vi "Motor_Open.vi"() -> ()   [LabVIEW 2016]
uses:
  <vilib>/Rock Robotics/WPI/SafetyOutput/WPI_SafetyOutputConfigMenu.ctl
  <vilib>/Rock Robotics/SystemInterfaces/DIO/FPGA_DIOPWMChannel.ctl
  <vilib>/Rock Robotics/WPI/ThirdParty/CanMotor/TalonSRX/WPI_CANTalonSRX_APIControlMode.ctl
  Drive/RobotDriveOpen6MotorWithTalonSR.vi
  Drive/RobotDriveOpen6MotorWithTalonSRX.vi
  <vilib>/Rock Robotics/WPI/MotorControl/WPI_MotorControlOpen Talon.vi
panel:
  in  "Left Motor 1 Inverted":bool=TRUE
  in  "Left Motor 2 Inverted":bool=TRUE
  in  "Right Motor 1 Inverted":bool=TRUE
  in  "Right Motor 2 Inverted":bool=TRUE
  in  "Competition_Robot?":bool
  in  "Right Motor 3 Inverted":bool=TRUE
  in  "Right Motor 2 Inverted":bool=TRUE
  in  "Right Motor 1 Inverted":bool=TRUE
  in  "Left Motor 3 Inverted":bool=TRUE
  in  "Left Motor 2 Inverted":bool=TRUE
  in  "Left Motor 1 Inverted":bool=TRUE
  # "Can"
  # "PWM"
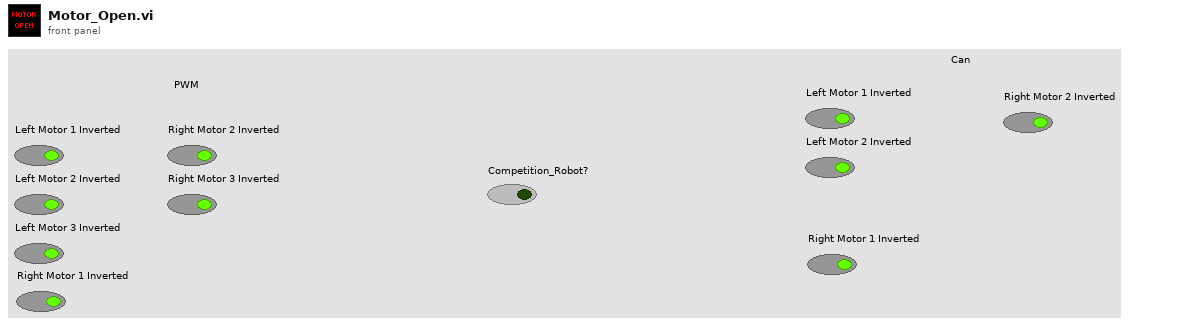
[diagram p1: front panel]
types:
  T1 = typedef "WPI_SafetyOutputConfigMenu.ctl" = enum16{"Enable", "Disable"}
  T2 = typedef "FPGA_DIOPWMChannel.ctl" = enum8{"PWM 0", "PWM 1", "PWM 2", "PWM 3", "PWM 4", "PWM 5", "PWM 6", "PWM 7", "PWM 8", "PWM 9", "PWM MXP 0", "PWM MXP 1", "PWM MXP 2", "PWM MXP 3", "PWM MXP 4", "PWM MXP 5", "PWM MXP 6", "PWM MXP 7", "PWM MXP 8", "PWM MXP 9", "Invalid"}
  T3 = typedef "WPI_CANTalonSRX_APIControlMode.ctl" = enum8{"Percent VBus", "Speed", "Position", "Slave", "Unchanged / Invalid", "Voltage Compensation", "Current", "Motion Profile", "Motion Magic"}
  T4 = typedef "WPI_RobotDriveDevRef.ctl" = cluster{"DevStatus":errorcluster, "Motors[]":T5[], "Square Inputs":bool, "Max Output":dbl}
  T5 = typedef "WPI_MotorControlDeviceRef.ctl" = cluster{"DeviceStatus":errorcluster, "Type":T6, "PWM":cluster{"PWM Channel":T2, "DeadBand":T7}, "CAN":cluster{"Device Number":u8, "SetOutput VI Ref":variant, "GetOutput VI Ref":variant, "Enable VI Ref":variant, "Disable VI Ref":variant, "Data":variant}, "Invert":bool}
  T6 = typedef "WPI_MotorControlType.ctl" = enum16{"PWM", "CAN"}
  T7 = typedef "WPI_PWMDeadband.ctl" = cluster{"Name":string, "maxPositivePwm":i32, "minPositivePwm":i32, "centerPwm":i32, "maxNegativePwm":i32, "minNegativePwm":i32, "angularRange":u16}
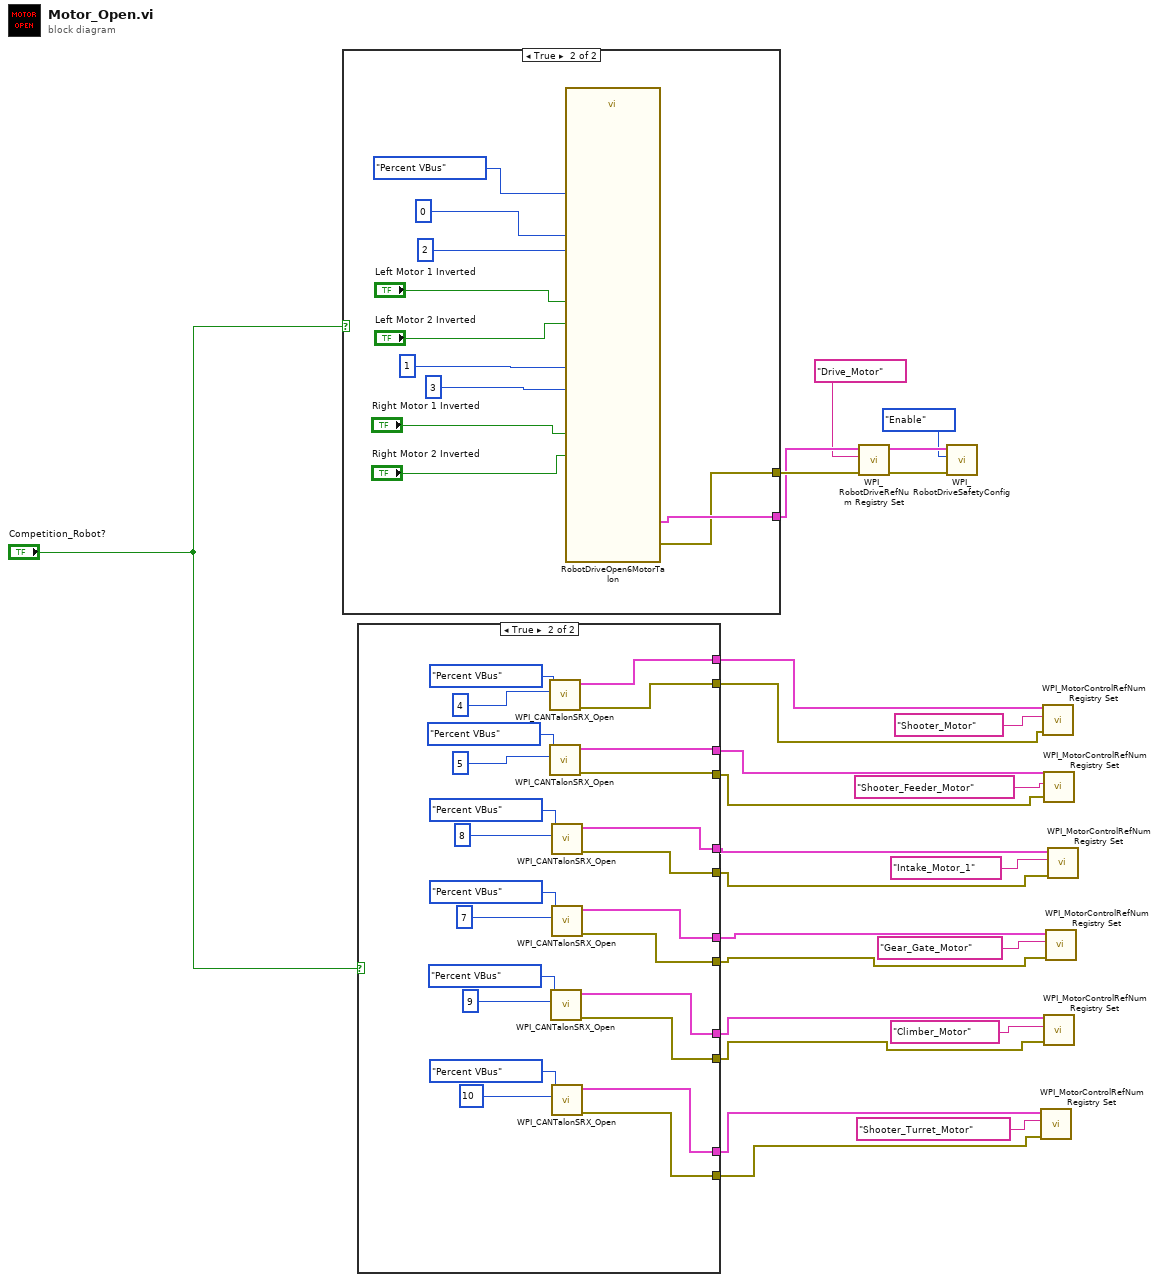
[diagram p0: block diagram]
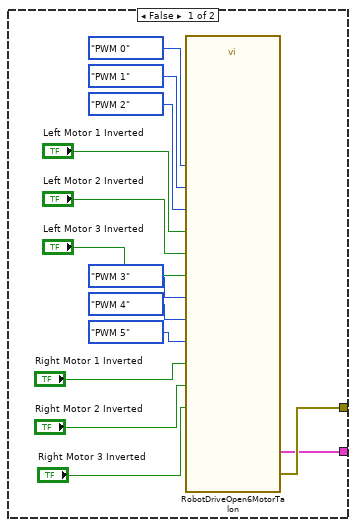
[diagram p2: hidden frame]
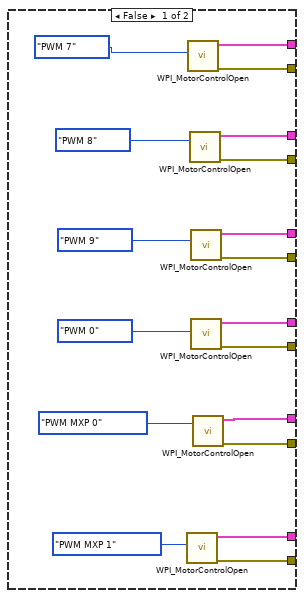
[diagram p3: hidden frame]
diagram:
  n1 = case shown="True" "Competition_Robot?" {
    tunnel: [w33 w45] -> w25
    tunnel: [w32 w46] -> w24
    frame False {
      n2 = call-poly "RobotDriveOpen6MotorTalon.vi"("Left Motor 1"=FPGA_DIOPWMChannel."PWM 0", "Left Motor 2"=FPGA_DIOPWMChannel."PWM 1", "Left Motor 3"=FPGA_DIOPWMChannel."PWM 2", "Right Motor 1"=FPGA_DIOPWMChannel."PWM 3", "Right Motor 2"=FPGA_DIOPWMChannel."PWM 4", "Right Motor 3"=FPGA_DIOPWMChannel."PWM 5", "Left Motor 1 Inverted"="Left Motor 1 Inverted", "Right Motor 1 Inverted"="Right Motor 1 Inverted", "Left Motor 2 Inverted"="Left Motor 2 Inverted", "Right Motor 2 Inverted"="Right Motor 2 Inverted", "Left Motor 3 Inverted"="Left Motor 3 Inverted", "Right Motor 3 Inverted"="Right Motor 3 Inverted") -> ("RobotDriveDevRef"=w32:T4, "error out"=w33:errorcluster)  [unwired: 14 in]
    }
    frame True {
      n3 = call-poly "RobotDriveOpen6MotorTalon.vi"("Left Motor 1"=u8 0, "Left Motor 2"=u8 2, "Right Motor 1"=u8 1, "Right Motor 2"=u8 3, "Left Motor 1 Inverted"="Left Motor 1 Inverted", "Right Motor 1 Inverted"="Right Motor 1 Inverted", "Left Motor 2 Inverted"="Left Motor 2 Inverted", "Right Motor 2 Inverted"="Right Motor 2 Inverted", "Control Mode"=WPI_CANTalonSRX_APIControlMode."Percent VBus") -> ("RobotDriveDevRef"=w46:T4, "error out"=w45:errorcluster)  [unwired: 17 in]
    }
  }
  n4 = case shown="True" "Competition_Robot?" {
    tunnel: [w62 w80] -> w13
    tunnel: [w61 w79] -> w12
    tunnel: [w60 w78] -> w11
    tunnel: [w59 w77] -> w10
    tunnel: [w58 w76] -> w9
    tunnel: [w57 w75] -> w8
    tunnel: [w56 w74] -> w7
    tunnel: [w55 w73] -> w6
    tunnel: [w54 w72] -> w5
    tunnel: [w53 w71] -> w4
    tunnel: [w52 w70] -> w3
    tunnel: [w51 w69] -> w2
    frame False {
      n5 = call-poly <vilib>:"WPI_MotorControlOpen.vi"("PWM Channel"=FPGA_DIOPWMChannel."PWM MXP 1") -> ("error out"=w51:errorcluster, "MotorControlDeviceRef"=w52:T5)  [unwired: 9 in]
      n6 = call-poly <vilib>:"WPI_MotorControlOpen.vi"("PWM Channel"=FPGA_DIOPWMChannel."PWM 7") -> ("error out"=w61:errorcluster, "MotorControlDeviceRef"=w62:T5)  [unwired: 9 in]
      n7 = call-poly <vilib>:"WPI_MotorControlOpen.vi"("PWM Channel"=FPGA_DIOPWMChannel."PWM 8") -> ("error out"=w59:errorcluster, "MotorControlDeviceRef"=w60:T5)  [unwired: 9 in]
      n8 = call-poly <vilib>:"WPI_MotorControlOpen.vi"("PWM Channel"=FPGA_DIOPWMChannel."PWM 9") -> ("error out"=w57:errorcluster, "MotorControlDeviceRef"=w58:T5)  [unwired: 9 in]
      n9 = call-poly <vilib>:"WPI_MotorControlOpen.vi"("PWM Channel"=FPGA_DIOPWMChannel."PWM 0") -> ("error out"=w55:errorcluster, "MotorControlDeviceRef"=w56:T5)  [unwired: 9 in]
      n10 = call-poly <vilib>:"WPI_MotorControlOpen.vi"("PWM Channel"=FPGA_DIOPWMChannel."PWM MXP 0") -> ("error out"=w53:errorcluster, "MotorControlDeviceRef"=w54:T5)  [unwired: 9 in]
    }
    frame True {
      n11 = call <vilib>:"WPI_CANTalonSRX_Open.vi"("Device Number"=u8 4, "Control Mode"=WPI_CANTalonSRX_APIControlMode."Percent VBus") -> ("error out"=w79:errorcluster, "CAN Talon SRX Ref"=w80:T5)  [unwired: 8 in]
      n12 = call <vilib>:"WPI_CANTalonSRX_Open.vi"("Device Number"=u8 5, "Control Mode"=WPI_CANTalonSRX_APIControlMode."Percent VBus") -> ("error out"=w77:errorcluster, "CAN Talon SRX Ref"=w78:T5)  [unwired: 8 in]
      n13 = call <vilib>:"WPI_CANTalonSRX_Open.vi"("Device Number"=u8 9, "Control Mode"=WPI_CANTalonSRX_APIControlMode."Percent VBus") -> ("error out"=w71:errorcluster, "CAN Talon SRX Ref"=w72:T5)  [unwired: 8 in]
      n14 = call <vilib>:"WPI_CANTalonSRX_Open.vi"("Device Number"=u8 8, "Control Mode"=WPI_CANTalonSRX_APIControlMode."Percent VBus") -> ("error out"=w75:errorcluster, "CAN Talon SRX Ref"=w76:T5)  [unwired: 8 in]
      n15 = call <vilib>:"WPI_CANTalonSRX_Open.vi"("Device Number"=u8 7, "Control Mode"=WPI_CANTalonSRX_APIControlMode."Percent VBus") -> ("error out"=w73:errorcluster, "CAN Talon SRX Ref"=w74:T5)  [unwired: 8 in]
      n16 = call <vilib>:"WPI_CANTalonSRX_Open.vi"("Device Number"=u8 10, "Control Mode"=WPI_CANTalonSRX_APIControlMode."Percent VBus") -> ("error out"=w69:errorcluster, "CAN Talon SRX Ref"=w70:T5)  [unwired: 8 in]
    }
  }
  n17 = call <vilib>:"WPI_RobotDriveRefNum Registry Set.vi"("error in (no error)"=w25, "refnum name"="Drive_Motor", "RobotDriveDevRef"=w24) -> ("error out"=w22:errorcluster, "RobotDriveDevRef"=w23:T4)  [unwired: 7 in]
  n18 = call <vilib>:"WPI_RobotDriveSafetyConfig.vi"("error in (no error)"=w22, "mode"=WPI_SafetyOutputConfigMenu."Enable", "RobotDriveDevRef"=w23) -> ()  [unwired: 7 in, 2 out]
  n19 = call <vilib>:"WPI_MotorControlRefNum Registry Set.vi"("error in (no error)"=w2, "refnum name"="Shooter_Turret_Motor", "MotorControlDevRef"=w3) -> ()  [unwired: 7 in, 2 out]
  n20 = call <vilib>:"WPI_MotorControlRefNum Registry Set.vi"("error in (no error)"=w12, "refnum name"="Shooter_Motor", "MotorControlDevRef"=w13) -> ()  [unwired: 7 in, 2 out]
  n21 = call <vilib>:"WPI_MotorControlRefNum Registry Set.vi"("error in (no error)"=w10, "refnum name"="Shooter_Feeder_Motor", "MotorControlDevRef"=w11) -> ()  [unwired: 7 in, 2 out]
  n22 = call <vilib>:"WPI_MotorControlRefNum Registry Set.vi"("error in (no error)"=w4, "refnum name"="Climber_Motor", "MotorControlDevRef"=w5) -> ()  [unwired: 7 in, 2 out]
  n23 = call <vilib>:"WPI_MotorControlRefNum Registry Set.vi"("error in (no error)"=w6, "refnum name"="Gear_Gate_Motor", "MotorControlDevRef"=w7) -> ()  [unwired: 7 in, 2 out]
  n24 = call <vilib>:"WPI_MotorControlRefNum Registry Set.vi"("error in (no error)"=w8, "refnum name"="Intake_Motor_1", "MotorControlDevRef"=w9) -> ()  [unwired: 7 in, 2 out]
